vi "unpack20bytes.vi"(7 "Reserved":u16[](array[numeric])=[0, 0, 0, 1] format="%x") -> (4 "number":u32, 6 "number 2":u32, 8 "number 3":u32, 10 "number 4":u32, 15 "number 5":u32)   [LabVIEW 2020]
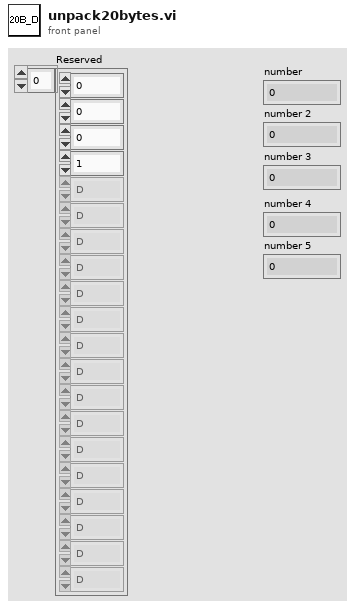
[diagram p1: front panel]
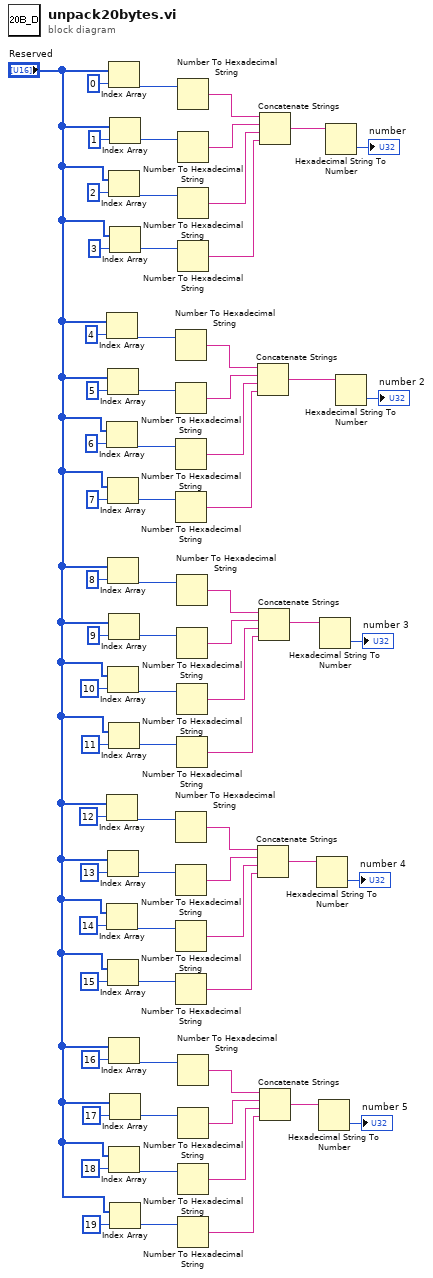
[diagram p0: block diagram]
diagram:
  n1 = Index Array(array="Reserved", index=4) -> (element=w56:u16)
  n2 = Index Array(array="Reserved", index=6) -> (element=w50:u16)
  n3 = Index Array(array="Reserved", index=12) -> (element=w32:u16)
  n4 = Index Array(array="Reserved", index=14) -> (element=w26:u16)
  n5 = Index Array(array="Reserved", index=5) -> (element=w55:u16)
  n6 = Index Array(array="Reserved", index=7) -> (element=w49:u16)
  n7 = Index Array(array="Reserved", index=8) -> (element=w44:u16)
  n8 = Index Array(array="Reserved", index=10) -> (element=w38:u16)
  n9 = Index Array(array="Reserved", index=13) -> (element=w31:u16)
  n10 = Index Array(array="Reserved", index=15) -> (element=w25:u16)
  n11 = Index Array(array="Reserved", index=0) -> (element=w69:u16)
  n12 = Index Array(array="Reserved", index=2) -> (element=w62:u16)
  n13 = Index Array(array="Reserved", index=9) -> (element=w43:u16)
  n14 = Index Array(array="Reserved", index=11) -> (element=w37:u16)
  n15 = Index Array(array="Reserved", index=16) -> (element=w20:u16)
  n16 = Index Array(array="Reserved", index=18) -> (element=w14:u16)
  n17 = Index Array(array="Reserved", index=1) -> (element=w68:u16)
  n18 = Index Array(array="Reserved", index=3) -> (element=w61:u16)
  n19 = Index Array(array="Reserved", index=17) -> (element=w19:u16)
  n20 = Index Array(array="Reserved", index=19) -> (element=w13:u16)
  n21 = Number To Hexadecimal String(2:w56) -> (0:w54:string)  [unwired: 1 in]
  n22 = Number To Hexadecimal String(2:w55) -> (0:w53:string)  [unwired: 1 in]
  n23 = Number To Hexadecimal String(2:w50) -> (0:w48:string)  [unwired: 1 in]
  n24 = Number To Hexadecimal String(2:w49) -> (0:w47:string)  [unwired: 1 in]
  n25 = Number To Hexadecimal String(2:w32) -> (0:w30:string)  [unwired: 1 in]
  n26 = Number To Hexadecimal String(2:w31) -> (0:w29:string)  [unwired: 1 in]
  n27 = Number To Hexadecimal String(2:w26) -> (0:w24:string)  [unwired: 1 in]
  n28 = Number To Hexadecimal String(2:w25) -> (0:w23:string)  [unwired: 1 in]
  n29 = Number To Hexadecimal String(2:w44) -> (0:w42:string)  [unwired: 1 in]
  n30 = Number To Hexadecimal String(2:w43) -> (0:w41:string)  [unwired: 1 in]
  n31 = Number To Hexadecimal String(2:w38) -> (0:w36:string)  [unwired: 1 in]
  n32 = Number To Hexadecimal String(2:w37) -> (0:w35:string)  [unwired: 1 in]
  n33 = Number To Hexadecimal String(2:w69) -> (0:w67:string)  [unwired: 1 in]
  n34 = Number To Hexadecimal String(2:w68) -> (0:w66:string)  [unwired: 1 in]
  n35 = Number To Hexadecimal String(2:w62) -> (0:w60:string)  [unwired: 1 in]
  n36 = Number To Hexadecimal String(2:w61) -> (0:w59:string)  [unwired: 1 in]
  n37 = Number To Hexadecimal String(2:w20) -> (0:w18:string)  [unwired: 1 in]
  n38 = Number To Hexadecimal String(2:w19) -> (0:w17:string)  [unwired: 1 in]
  n39 = Number To Hexadecimal String(2:w14) -> (0:w12:string)  [unwired: 1 in]
  n40 = Number To Hexadecimal String(2:w13) -> (0:w11:string)  [unwired: 1 in]
  n41 = Concatenate Strings(w54, w53, w48, w47) -> (w10:string)
  n42 = Concatenate Strings(w30, w29, w24, w23) -> (w8:string)
  n43 = Concatenate Strings(w42, w41, w36, w35) -> (w9:string)
  n44 = Concatenate Strings(w67, w66, w60, w59) -> (w65:string)
  n45 = Concatenate Strings(w18, w17, w12, w11) -> (w7:string)
  n46 = Hexadecimal String To Number(string=w8) -> (number=→"number 4":u32)  [unwired: 2 in, 1 out]
  n47 = Hexadecimal String To Number(string=w7) -> (number=→"number 5":u32)  [unwired: 2 in, 1 out]
  n48 = Hexadecimal String To Number(string=w9) -> (number=→"number 3":u32)  [unwired: 2 in, 1 out]
  n49 = Hexadecimal String To Number(string=w65) -> (number=→"number":u32)  [unwired: 2 in, 1 out]
  n50 = Hexadecimal String To Number(string=w10) -> (number=→"number 2":u32)  [unwired: 2 in, 1 out]
